vi "ReadTSVariables.vi"(8 "error in (no error)":errorcluster, 11 "Automation Refnum in":refnum<k7>) -> (0 "error out":errorcluster, 2 "FirmwareVersion":string, 3 "Url":string)   [LabVIEW 2021]
uses:
  <vilib>/addons/TestStand/_TSUtility.llb/TestStand - Get Property Value (String).vi
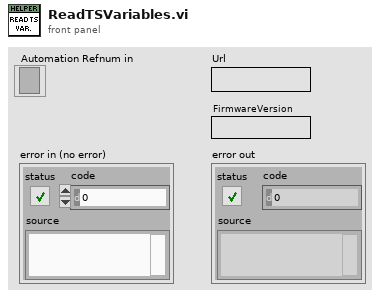
[diagram p1: front panel]
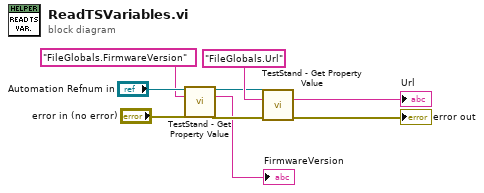
[diagram p0: block diagram]
diagram:
  n1 = call-poly <vilib>:"TestStand - Get Property Value.vi"("Sequence Context In"="Automation Refnum in", "Lookup String"="FileGlobals.FirmwareVersion", "error in (no error)"="error in (no error)") -> ("Sequence Context Out"=w5:refnum<k7>, "Value"=→"FirmwareVersion":string, "error out"=w3:errorcluster)  [unwired: 10 in]
  n2 = call-poly <vilib>:"TestStand - Get Property Value.vi"("Sequence Context In"=w5, "Lookup String"="FileGlobals.Url", "error in (no error)"=w3) -> ("Value"=→"Url":string, "error out"=→"error out":errorcluster)  [unwired: 10 in, 1 out]
